vi "DriveGlobal.vi"() -> ()   [LabVIEW 2023]
doc: "Global variables for drive"
uses:
  <vilib>/Rock Robotics/WPI/ThirdParty/JAS_Junk/TrajLib/TypeDef/CHASSIS_SPEEDS.ctl
  <vilib>/Rock Robotics/WPI/ThirdParty/JAS_Junk/TrajLib/TypeDef/SWERVE_DRIVE_KINEMATICS.ctl
  <vilib>/Analysis/Matrix/Datatypes/RealMatrix.ctl
  <vilib>/Rock Robotics/WPI/ThirdParty/JAS_Junk/TrajLib/TypeDef/TRANSLATION2D.ctl
  <vilib>/Rock Robotics/WPI/ThirdParty/JAS_Junk/TrajLib/TypeDef/SWERVE_DRIVE_MODULE_STATE.ctl
  <vilib>/Rock Robotics/WPI/ThirdParty/JAS_Junk/TrajLib/TypeDef/ROTATION2D.ctl
  <vilib>/Rock Robotics/WPI/ThirdParty/JAS_Junk/TrajLib/TypeDef/SWERVE_DRIVE_MODULE_POSITION.ctl
  <vilib>/Rock Robotics/WPI/ThirdParty/JAS_Junk/TrajLib/Trajectory_Library.lvlib
  <vilib>/Analysis/Matrix/NI_Matrix.lvlib
panel:
  out "SpdDmd_Rate_Limit_Enable":bool=TRUE
  out "SpdDmd_Y_Rate_Limit_M/SS":dbl=40.0
  out "SpdDmd_X_Rate_Limt_M/SS":dbl=40.0
  out "ModuleSpinPosDmd":dbl[](array[numeric])
  out "ModuleSpinMotorDmd":dbl[](array[numeric])
  out "ModuleSpinPosErr":dbl[](array[numeric])
  out "ModuleTravelMotorDmd":dbl[](array[numeric])
  out "ModuleTravelVelocityErr":dbl[](array[numeric])
  out "ModuleTravelVelocityDmd":dbl[](array[numeric])
  out "Gyro YawModulu":dbl
  in  "GyroYawRotation":T1={"VALUE"=0.0, "COS"=1.0, "SIN"=0.0} {"SIN" format="%13.4f"; "COS" format="%13.4f"; "VALUE" format="%13.4f"}
  out "Swerve_Drive_Modual_Position":T2[](array[typedef]) {"Angle"."SIN" format="%13.4f"; "Angle"."COS" format="%13.4f"; "Angle"."VALUE" format="%13.4f"}
  out "Swerve__Drive_Modual_States":T3[](array[typedef]) {"Angle"."SIN" format="%13.4f"; "Angle"."COS" format="%13.4f"; "Angle"."VALUE" format="%13.4f"}
  out "RobotInitialOrientationDeg":dbl=180.0
  out "ModuleEncoderAbsPosition":dbl[](array[numeric])
  out "ModuleSpinVelocity":dbl[](array[numeric])
  out "ModuleSpinPosition":dbl[](array[numeric])
  out "ModuleTravelVelocity":dbl[](array[numeric])
  out "ModuleTravelPosition":dbl[](array[numeric])
  out "SWERVE_DRIVE_KINEMATICS":T4 {"SavedModuleStates"."Angle"."SIN" format="%13.4f"; "SavedModuleStates"."Angle"."COS" format="%13.4f"; "SavedModuleStates"."Angle"."VALUE" format="%13.4f"; "PrevCoR"."Y" format="%14.3f"; "PrevCoR"."X" format="%14.3f"; "Modules"."Y" format="%14.3f"; "Modules"."X" format="%14.3f"}
  out "ChassisSpeedDemand":T7 {"vOmega" format="%10.3f"; "vY" format="%10.3f"; "vX" format="%10.3f"}
  out "GryoCalibrated":bool
  out "CalibrateGyro":bool
  out "SpeedModifer":dbl
  out "GyroYawZero":dbl
  out "Gyro Pitch":dbl
  out "Gyro YawRaw":dbl
  out "Gyro Roll":dbl
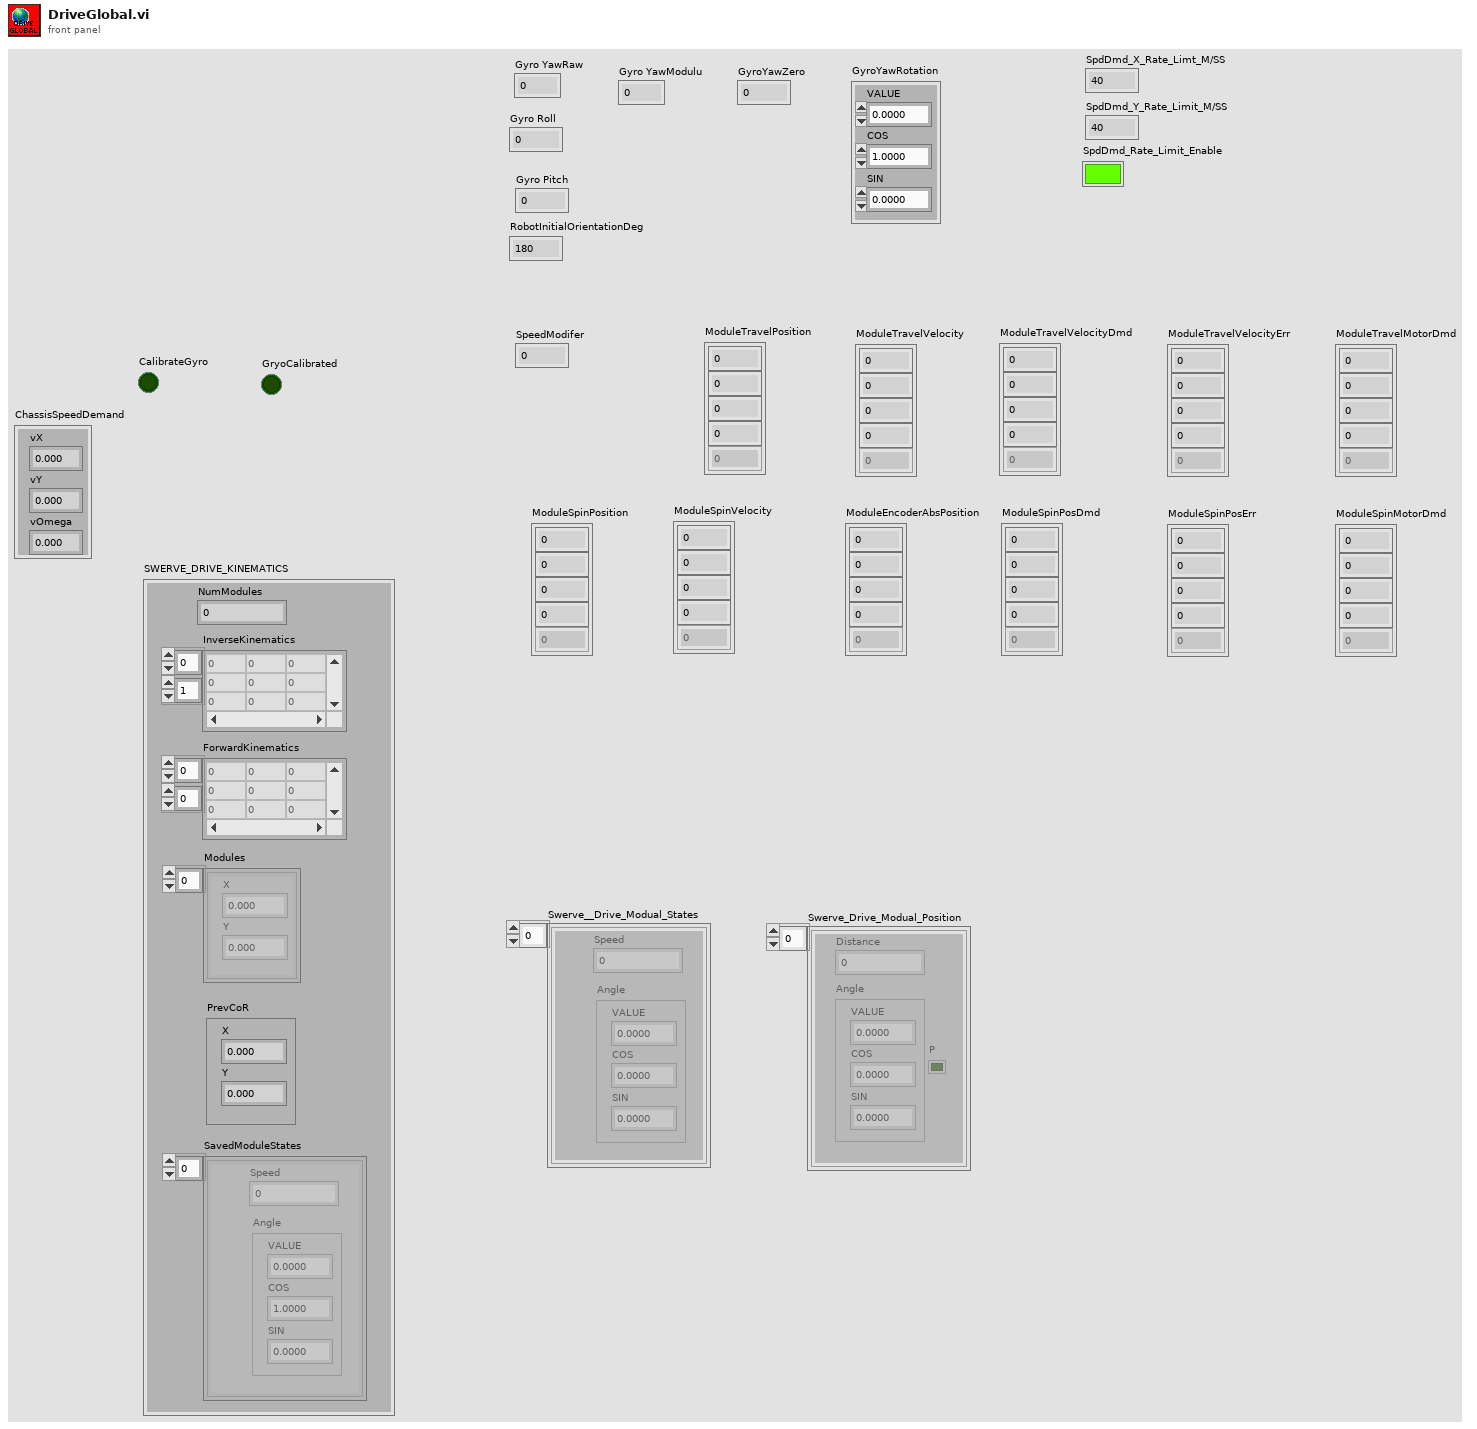
[diagram p1: front panel]
types:
  T1 = typedef "Trajectory_Library.lvlib/ROTATION2D.ctl" = cluster{"VALUE":dbl, "COS":dbl, "SIN":dbl}
  T2 = typedef "Trajectory_Library.lvlib/SWERVE_DRIVE_MODULE_POSITION.ctl" = cluster{"Distance":dbl, "Angle":T1, "P":bool}
  T3 = typedef "Trajectory_Library.lvlib/SWERVE_DRIVE_MODULE_STATE.ctl" = cluster{"Speed":dbl, "Angle":T1}
  T4 = typedef "Trajectory_Library.lvlib/SWERVE_DRIVE_KINEMATICS.ctl" = cluster{"NumModules":i32, "InverseKinematics":T5, "ForwardKinematics":T5, "Modules":T6[], "PrevCoR":T6, "SavedModuleStates":T3[]}
  T5 = typedef "NI_Matrix.lvlib/RealMatrix.ctl" = dbl[][]
  T6 = typedef "Trajectory_Library.lvlib/TRANSLATION2D.ctl" = cluster{"X":dbl, "Y":dbl}
  T7 = typedef "Trajectory_Library.lvlib/CHASSIS_SPEEDS.ctl" = cluster{"vX":dbl, "vY":dbl, "vOmega":dbl}
diagram:
